vi "Controller Configuration Loop.vi"(7 "Sync Objects":T1, 8 "error in (no error)":errorcluster, 11 "FOFB Configuration":T4={"FOFB Parameters"={"Network"={"FOFB Controller IP"="", "LNLS Control Network IP"="", "LNLS Control Network Power Supplies TCP Port"=0, "LNLS Control Network FOFB Configuration TCP Port"=0, "LNLS Control Network BPMs TCP Port"=0, "Data Server TCP Port"=0, "Monitoring Data TCP Port"=0, "Configuration GUI TCP Port"=0, "Storage Data TCP Port"=0, "Fast Command TCP Port"=0, "TCP Listening Timeout"=0, "Request Setpoints Rate"=0}, "Fast Acquisition"={"Acquisition Period"=0, "Data Buffer Size"=0, "Monitoring Period"=0}, "Response Matrix Measurement"={"Step Amplitude"=0.0, "Time Between Steps"=0, "Step Duration"=0, "Number of Averages"=0}, "Correction Algorithm"={"Correction Period"=0, "Reference Orbit Path"=path "", "Response Matrix Path"=path "", "Correction Matrix Path"=path "", "PID Horizontal Gain"=0.0, "PID Vertical Gain"=0.0, "PID Horizontal Integral Time"=0.0, "PID Vertical Integral Time"=0.0, "PID Horizontal Derivative Time"=0.0, "PID Vertical Derivative Time"=0.0, "Beam Current FOFB Threshold"=0.0, "Decouple H-V"=FALSE, "Use Additional BPM LPF"=FALSE, "BPM LPF Cutoff"=0.0}, "Acquisition Network"=[], "Actuation Network"=[]}, "Number of Acquisition Chassis"=0, "Number of Actuation Chassis"=0, "Number of BPM Readings"=0, "BPM Reading Names"=[], "Selected BPM Readings"=[0, 1, 2, 3, 4, 5, 6, 7, 8, 9, 10, 11, 12, 13, 14, 15, 16, 17, 18, 19, 20, 21, 22, 23, 24, 25, 26, 27, 28, 29, 30, 31, 32, 33, 34, 35, 36, 37, 38, 39, 40, 41, 42, 43, 44, 45, 46, 47, 48, 49], "Number of Correctors"=0, "Corrector Names"=[], "Selected Correctors"=[0, 1, 2, 3, 4, 5, 6, 7, 8, 9, 10, 11, 12, 13, 14, 15, 16, 17, 18, 19, 20, 21, 22, 23, 24, 25, 26, 27, 28, 29, 30, 31, 32, 33, 34, 35, 36, 37, 38, 39, 40, 41, 42, 43, 44, 45, 46, 47, 48, 49], "Reference Orbit"=[], "Response Matrix"=[], "Correction Matrix"=[], "Acquisition Chassis Names"=[], "Actuation Chassis Names"=[], "Acquisition Variables"=[], "Actuation Variables"=[], "PS Matrix Mapping"=[], "Inverse PS Matrix Mapping"=[], "BPM Matrix Mapping"=[], "Inverse BPM Matrix Mapping"=[], "Response Matrix Beam Energy (MeV)"=0.0, "PID Parameters"=[], "BPM Planes"=[], "Corrector Planes"=[], "RMM Step Factor"=[]}) -> (0 "error out":errorcluster)   [LabVIEW 2011, in "Controller VIs.lvlib"]
uses:
  Controller VIs.lvlib
  Types Definitions/Type FOFB Configuration.ctl
  Types Definitions/Type FOFB Parameters.ctl
  Types Definitions/Type Network Configuration.ctl
  Types Definitions/Type FA Configuration.ctl
  Types Definitions/Type Response Matrix Measurement Configuration.ctl
  Types Definitions/Type Correction Algorithm Configuration.ctl
  Types Definitions/Type Acquisition Network Configuration.ctl
  Types Definitions/Type Actuation Network Configuration.ctl
  Types Definitions/Type PID Parameters.ctl
  Types Definitions/Type Synchronization Objects.ctl
  Types Definitions/Type Blocking Synchronization Objects.ctl
  Types Definitions/Type Monitoring Data.ctl
  Types Definitions/Type Operation Mode State.ctl
  Types Definitions/Type Diagnostics Data.ctl
  Types Definitions/Type CPU Loads Array.ctl
  Types Definitions/Type CPU Loads.ctl
  Types Definitions/Type Non-blocking Synchronization Objects.ctl
  Types Definitions/Type FOFB Variables.ctl
  Types Definitions/Type Actuation State.ctl
  Types Definitions/Type TCP State.ctl
  <vilib>/Platform/TimedLoop/XDataNode/timing_clust.ctl
  <vilib>/Platform/TimedLoop/XDataNode/nitl_modes.ctl
  <vilib>/Platform/TimedLoop/XDataNode/wakeup.ctl
  Types Definitions/Type Configuration Data (GUI to Controller).ctl
  Controller Global Variables/LNLS Control FOFB Configuration In.vi
  <vilib>/Platform/TimedLoop/XDataNode/XDataNode.xnode
  Type Definitions.lvlib
  <vilib>/Platform/TimedLoop/XDataNode/XDNodeRunTimeDep.lvlib
  XML VIs.lvlib
  Controller Global Variables.lvlib
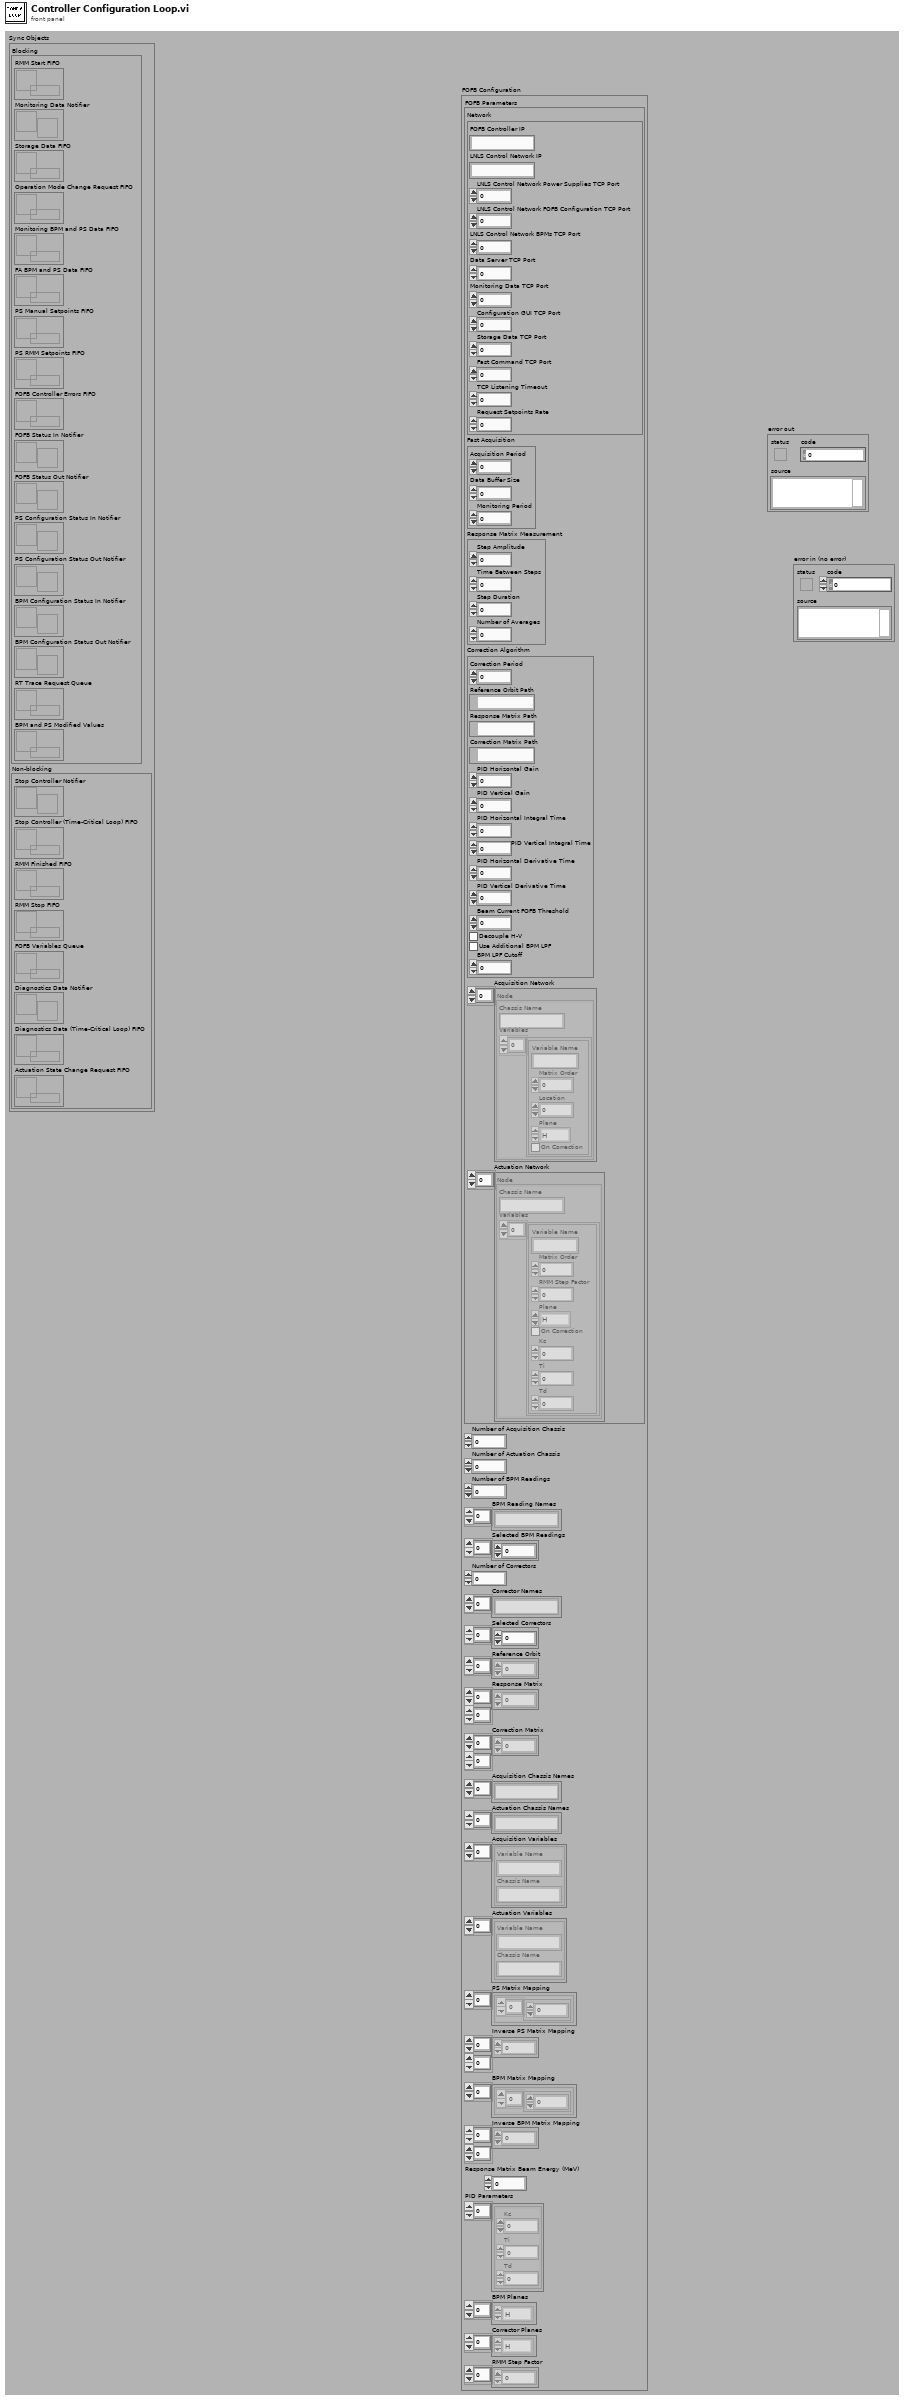
[diagram p1: front panel]
types:
  T1 = typedef "Type Definitions.lvlib/Type Synchronization Objects.ctl" = cluster{"Blocking":T2, "Non-blocking":T3}
  T2 = typedef "Type Definitions.lvlib/Type Blocking Synchronization Objects.ctl" = cluster{"RMM Start FIFO":refnum<k33>, "Monitoring Data Notifier":refnum<notifier>, "Storage Data FIFO":refnum<queue>, "Operation Mode Change Request FIFO":refnum<k33>, "Monitoring BPM and PS Data FIFO":refnum<k33>, "FA BPM and PS Data FIFO":refnum<k33>, "PS Manual Setpoints FIFO":refnum<k33>, "PS RMM Setpoints FIFO":refnum<k33>, "FOFB Controller Errors FIFO ":refnum<k33>, "FOFB Status In Notifier":refnum<notifier>, "FOFB Status Out Notifier":refnum<notifier>, "PS Configuration Status In Notifier":refnum<notifier>, "PS Configuration Status Out Notifier":refnum<notifier>, "BPM Configuration Status In Notifier":refnum<notifier>, "BPM Configuration Status Out Notifier":refnum<notifier>, "RT Trace Request Queue":refnum<queue>, "BPM and PS Modified Values":refnum<k33>}
  T3 = typedef "Type Definitions.lvlib/Type Non-blocking Synchronization Objects.ctl" = cluster{"Stop Controller Notifier":refnum<notifier>, "Stop Controller (Time-Critical Loop) FIFO":refnum<k33>, "RMM Finished FIFO":refnum<k33>, "RMM Stop FIFO":refnum<k33>, "FOFB Variables Queue":refnum<queue>, "Diagnostics Data Notifier":refnum<notifier>, "Diagnostics Data (Time-Critical Loop) FIFO":refnum<k33>, "Actuation State Change Request FIFO":refnum<k33>}
  T4 = typedef "Type Definitions.lvlib/Type FOFB Configuration.ctl" = cluster{"FOFB Parameters":T5, "Number of Acquisition Chassis":i32, "Number of Actuation Chassis":i32, "Number of BPM Readings":i32, "BPM Reading Names":string[], "Selected BPM Readings":u32[], "Number of Correctors":i32, "Corrector Names":string[], "Selected Correctors":u32[], "Reference Orbit":dbl[], "Response Matrix":dbl[][], "Correction Matrix":dbl[][], "Acquisition Chassis Names":string[], "Actuation Chassis Names":string[], "Acquisition Variables":cluster{"Variable Name":string, "Chassis Name":string}[], "Actuation Variables":cluster{"Variable Name":string, "Chassis Name":string}[], "PS Matrix Mapping":cluster{u32[]}[], "Inverse PS Matrix Mapping":u32[][], "BPM Matrix Mapping":cluster{u32[]}[], "Inverse BPM Matrix Mapping":u32[][], "Response Matrix Beam Energy (MeV)":dbl, "PID Parameters":T12[], "BPM Planes":enum8{"H", "V"}[], "Corrector Planes":enum8{"H", "V"}[], "RMM Step Factor":dbl[]}
  T5 = typedef "Type Definitions.lvlib/Type FOFB Parameters.ctl" = cluster{"Network":T6, "Fast Acquisition":T7, "Response Matrix Measurement":T8, "Correction Algorithm":T9, "Acquisition Network":T10, "Actuation Network":T11}
  T6 = typedef "Type Definitions.lvlib/Type Network Configuration.ctl" = cluster{"FOFB Controller IP":string, "LNLS Control Network IP":string, "LNLS Control Network Power Supplies TCP Port":u16, "LNLS Control Network FOFB Configuration TCP Port":u16, "LNLS Control Network BPMs TCP Port":u16, "Data Server TCP Port":u16, "Monitoring Data TCP Port":u16, "Configuration GUI TCP Port":u16, "Storage Data TCP Port":u16, "Fast Command TCP Port":u16, "TCP Listening Timeout":i32, "Request Setpoints Rate":u16}
  T7 = typedef "Type Definitions.lvlib/Type FA Configuration.ctl" = cluster{"Acquisition Period":u32, "Data Buffer Size":u32, "Monitoring Period":u32}
  T8 = typedef "Type Definitions.lvlib/Type Response Matrix Measurement Configuration.ctl" = cluster{"Step Amplitude":dbl, "Time Between Steps":u32, "Step Duration":u32, "Number of Averages":u32}
  T9 = typedef "Type Definitions.lvlib/Type Correction Algorithm Configuration.ctl" = cluster{"Correction Period":u32, "Reference Orbit Path":path, "Response Matrix Path":path, "Correction Matrix Path":path, "PID Horizontal Gain":dbl, "PID Vertical Gain":dbl, "PID Horizontal Integral Time":dbl, "PID Vertical Integral Time":dbl, "PID Horizontal Derivative Time":dbl, "PID Vertical Derivative Time":dbl, "Beam Current FOFB Threshold":dbl, "Decouple H-V":bool, "Use Additional BPM LPF":bool, "BPM LPF Cutoff":dbl}
  T10 = typedef "Type Definitions.lvlib/Type Acquisition Network Configuration.ctl" = cluster{"Chassis Name":string, "Variables":cluster{"Variable Name":string, "Matrix Order":u32, "Location":dbl, "Plane":enum8{"H", "V"}, "On Correction":bool}[]}[]
  T11 = typedef "Type Definitions.lvlib/Type Actuation Network Configuration.ctl" = cluster{"Chassis Name":string, "Variables":cluster{"Variable Name":string, "Matrix Order":u32, "RMM Step Factor":dbl, "Plane":enum8{"H", "V"}, "On Correction":bool, "Kc":dbl, "Ti":dbl, "Td":dbl}[]}[]
  T12 = typedef "Type Definitions.lvlib/Type PID Parameters.ctl" = cluster{"Kc":fxp<+/-,16,8>, "Ti":fxp<+/-,16,8>, "Td":fxp<+/-,16,8>}
  T13 = typedef "Type Definitions.lvlib/Type TCP State.ctl" = enum16{"Idle", "Wait Connection", "Read Data", "Process Data", "Write Data", "Close Connection"}
  T14 = typedef "XDNodeRunTimeDep.lvlib/timing_clust.ctl" = cluster{"Expected End [f-1]":u64, "Actual End [f-1]":u64, "Finished Late? [f-1]":bool, "Expected End [i-1]":u64, "Actual End [i-1]":u64, "Finished Late? [i-1]":bool, "Expected Start [i]":u64, "Actual Start [i]":u64, "Expected Start [f]":u64, "Actual Start [f]":u64, "Source Name":string, "Structure Name":string, "Period":i64, "Deadline":i64, "Offset":i64, "Start":i64, "Priority":i32, "Timeout":i32, "Mode":T15, "Wakeup Reason":T16, "Error":errorcluster, "Source Type":string, "Secondary Source Type":string, "Global End Time":u64, "Global Start Time":u64, "Frame Duration":u64, "Iteration Duration":u64, "Assigned CPU":i32, "I/O Scan Engine Mode":u32}
  T15 = typedef "XDNodeRunTimeDep.lvlib/nitl_modes.ctl" = enum32{"No Change", "Process missed periods, maintain original phase", "Discard missed periods, maintain original phase", "Process missed periods, ignore original phase", "Discard missed periods, ignore original phase"}
  T16 = typedef "XDNodeRunTimeDep.lvlib/wakeup.ctl" = enum32{"Normal", "Aborted", "Asynchronous wakeup", "Timing source error", "Timed loop error", "Timeout"}
  T17 = typedef "Type Definitions.lvlib/Type Configuration Data (GUI to Controller).ctl" = cluster{"Update Controller Soft Configuration":bool[], "Request RT Execution Trace":string[], "Reference Orbit":dbl[], "Request Response Matrix Folder List":bool[], "Request FOFB Parameters":bool[], "FOFB Parameters":T5[]}
  T18 = typedef "Type Definitions.lvlib/Type Configuration Change Acknowledge (Controller to GUI).ctl" = cluster{"Request Response Matrix List Folder":string[], "FOFB Parameters":T5[]}
  T19 = typedef "Type Definitions.lvlib/Type Control FOFB Configuration In.ctl" = cluster{"Status":u16, "Operation Mode":T20, "PID Horizontal Gain":sgl, "PID Vertical Gain":sgl, "PID Horizontal Integral Time":sgl, "PID Vertical Integral Time":sgl, "PID Horizontal Derivative Time":sgl, "PID Vertical Derivative Time":sgl, "Fast Command Enabled":bool}
  T20 = typedef "Type Definitions.lvlib/Type Operation Mode State.ctl" = enum8{"Idle Mode", "Manual Mode", "FOFB Mode", "RMM Mode"}
  T21 = cluster{"PID Horizontal Gain":sgl, "PID Vertical Gain":sgl, "PID Horizontal Integral Time":sgl, "PID Vertical Integral Time":sgl, "PID Horizontal Derivative Time":sgl, "PID Vertical Derivative Time":sgl, "Fast Command Enabled":bool}
  T22 = typedef "Type Definitions.lvlib/Type FOFB Variables.ctl" = cluster{"Correction Period":u32, "Reference Orbit":dbl[], "Response Matrix":dbl[][], "Correction Matrix":dbl[][], "Decouple H-V":bool, "PID Horizontal Gain":dbl, "PID Vertical Gain":dbl, "PID Horizontal Integral Time":dbl, "PID Vertical Integral Time":dbl, "PID Horizontal Derivative Time":dbl, "PID Vertical Derivative Time":dbl, "Selected BPM Readings":u32[], "Selected Correctors":u32[], "BPM Planes":enum8{"H", "V"}[], "Corrector Planes":enum8{"H", "V"}[], "Beam Current FOFB Threshold":dbl, "Response Matrix Beam Energy (MeV)":dbl, "Fast Command Enabled":bool}
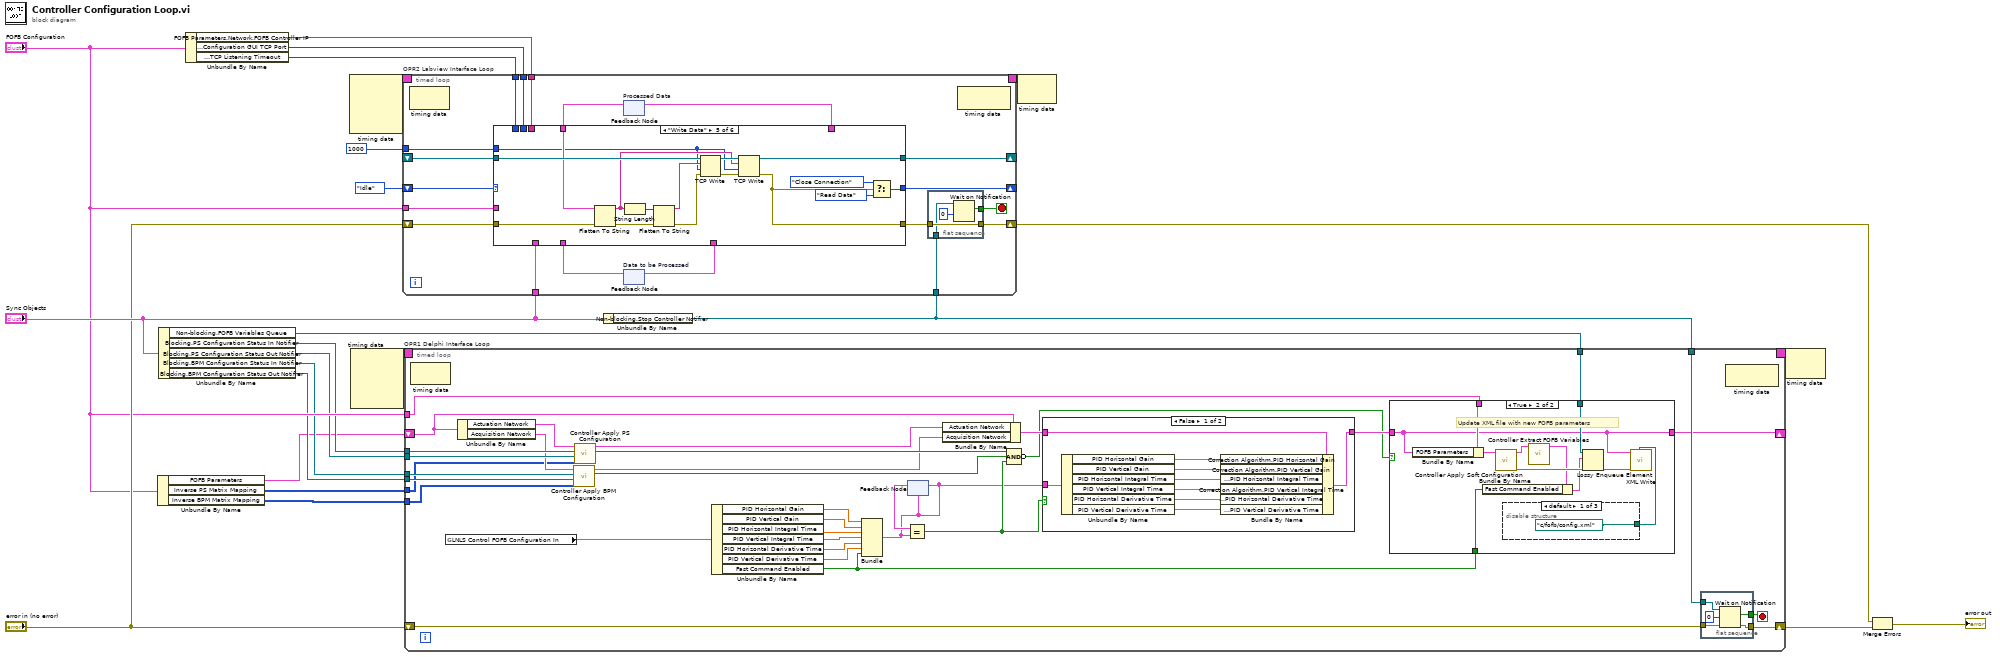
[diagram p0: block diagram]
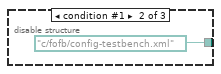
[diagram p4: hidden frame]
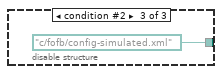
[diagram p5: hidden frame]
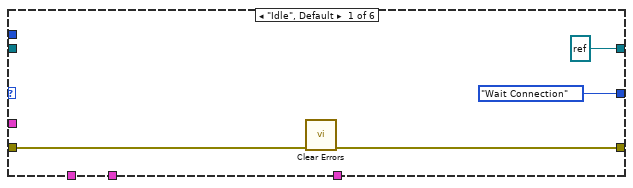
[diagram p6: hidden frame]
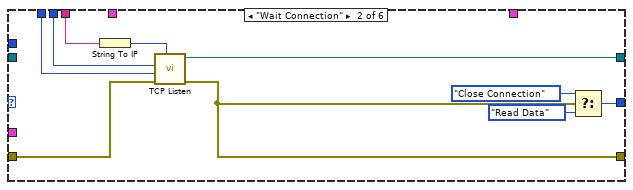
[diagram p7: hidden frame]
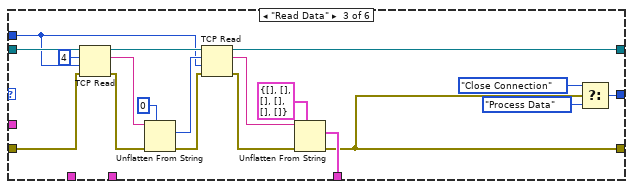
[diagram p8: hidden frame]
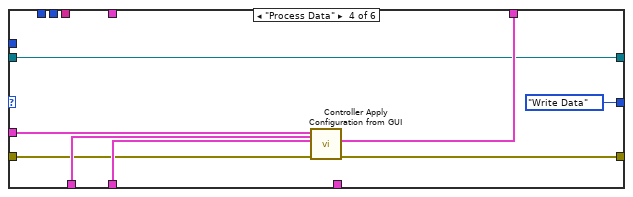
[diagram p9: hidden frame]
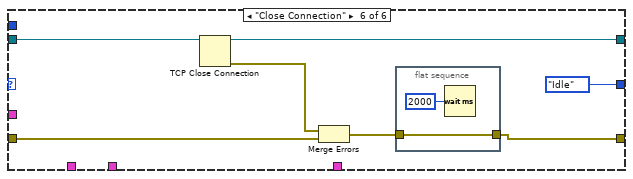
[diagram p10: hidden frame]
diagram:
  n1 = Unbundle By Name("FOFB Configuration") -> ("FOFB Parameters"=w4:T5, "Inverse PS Matrix Mapping"=w3:u32[][], "Inverse BPM Matrix Mapping"=w2:u32[][])
  n2 = Unbundle By Name("Sync Objects") -> ("Non-blocking.FOFB Variables Queue"=w9:refnum<queue>, "Blocking.PS Configuration Status In Notifier"=w7:refnum<notifier>, "Blocking.PS Configuration Status Out Notifier"=w6:refnum<notifier>, "Blocking.BPM Configuration Status In Notifier"=w8:refnum<notifier>, "Blocking.BPM Configuration Status Out Notifier"=w5:refnum<notifier>)
  n3 = Unbundle By Name("FOFB Configuration") -> ("FOFB Parameters.Network.FOFB Controller IP"=w24:string, "FOFB Parameters.Network.Configuration GUI TCP Port"=w22:u16, "FOFB Parameters.Network.TCP Listening Timeout"=w23:i32)
  n4 = node-c288() -> (w21:T14)  [unwired: 4 in]
  n5 = node-c288() -> (w11:T14)  [unwired: 4 in]
  n6 = Unbundle By Name("Sync Objects") -> ("Non-blocking.Stop Controller Notifier"=w17:refnum<notifier>)
  n7 = timed-loop "OPR2 Labview Interface Loop" {
    tunnel: w24 -> [w43]
    tunnel: w22 -> [w42]
    tunnel: w23 -> [w41]
    shift-right: [w29] -> w15
    shift-left: "error in (no error)" -> [w38]
    shift-right: [w36] -> _
    shift-left: Type_TCP_State."Idle" ("f") -> [w37]
    shift-right: [w39] -> _
    shift-left: _ -> [w40]
    tunnel: w17 -> [w28]
    tunnel: "Sync Objects" -> [w33]
    timing: w21 -> [_]
    timing-out: [_] -> w20
    tunnel: "FOFB Configuration" -> [w26]
    tunnel: 1000 ("TCP Listening Timeout") -> [w25]
    stop <- w27 stop-if-true
    n8 = node-c288() -> ()  [unwired: 1 in, 1 out]
    n9 = feedback #1 "Processed Data"() -> (w32:T18)  [unwired: 1 in]
    n10 = feedback #2 "Data to be Processed"() -> (w34:T17)  [unwired: 1 in]
    n11 = case shown="\"Write Data\"" w37 {
      tunnel: [refnum<k5> refnum ("connection ID") w63 w75 w89 w106 w113] -> w39
      tunnel: [Type_TCP_State."Wait Connection" ("f") w62 w71 Type_TCP_State."Write Data" ("f") w105 Type_TCP_State."Idle" ("f")] -> w36
      tunnel: [w50 w57 w67 w83 w104 w107] -> w30
      tunnel: w38 -> [w51 w56 w74 w84 w94 w109]
      tunnel: w40 -> [_ _ w76 w89 w102 w111]
      tunnel: w43 -> [_ w61 _ _ _ _]
      tunnel: w42 -> [_ w59 _ _ _ _]
      tunnel: w41 -> [_ w54 _ _ _ _]
      tunnel: [_ _ w69 _ _ _] -> w35
      tunnel: w34 -> [_ _ _ w86 _ _]
      tunnel: w33 -> [_ _ _ w87 _ _]
      tunnel: w32 -> [_ _ _ _ w95 _]
      tunnel: [_ _ _ w90 _ _] -> w31
      tunnel: w26 -> [_ _ _ w85 _ _]
      tunnel: w25 -> [_ _ w64 _ w91 _]
      frame "Idle", Default {
        n12 = call <vilib>:"Clear Errors.vi"("error in (no error)"=w51) -> ("error out"=w50:errorcluster)  [unwired: 6 in]
      }
      frame "Wait Connection" {
        n13 = String To IP(1:w61) -> (0:w60:u32)
        n14 = call <vilib>:"TCP Listen.vi"("net address"=w60, "error in (no error)"=w56, "timeout ms (wait forever: -1)"=w54, "port"=w59) -> ("error out"=w57:errorcluster, "connection ID"=w63:refnum<k5>)  [unwired: 3 in, 3 out]
        n15 = Select(t=Type_TCP_State."Close Connection" ("f"), s=w57, f=Type_TCP_State."Read Data") -> (s? t:f=w62:T13)
      }
      frame "Read Data" {
        n16 = TCP Read(connection ID=w76, bytes to read=4, error in (no error)=w74, 9:w64) -> (connection ID out=w82:refnum<k5>, data out=w80:string, error out=w66:errorcluster)  [unwired: 1 in]
        n17 = Unflatten From String(type=0 ("bytes to read"), binary string=w80, error in (no error)=w66) -> (value=w78:i32, error out=w68:errorcluster)  [unwired: 2 in, 1 out]
        n18 = TCP Read(connection ID=w82, bytes to read=w78, error in (no error)=w68, 9:w64) -> (connection ID out=w75:refnum<k5>, data out=w77:string, error out=w65:errorcluster)  [unwired: 1 in]
        n19 = Unflatten From String(type=T17 {"Update Controller Soft Configuration"=[], "Request RT Execution Trace"=[], "Reference Orbit"=[], "Request Response Matrix Folder List"=[], "Request FOFB Parameters"=[], "FOFB Parameters"=[]} ("Configuration Data (GUI to Controller)"), binary string=w77, error in (no error)=w65) -> (value=w69:T17, error out=w67:errorcluster)  [unwired: 2 in, 1 out]
        n20 = Select(t=Type_TCP_State."Close Connection" ("f"), s=w67, f=Type_TCP_State."Process Data") -> (s? t:f=w71:T13)
      }
      frame "Process Data" {
        n21 = call "Controller Apply Configuration from GUI.vi"("Sync Objects"=w87, "error in (no error)"=w84, "Configuration Data (GUI to Controller)"=w86, "FOFB Configuration"=w85) -> ("error out"=w83:errorcluster, "Configuration Change Acknowledge (Controller to GUI)"=w90:T18)  [unwired: 6 in]
      }
      frame "Write Data" {
        n22 = Flatten To String(anything=w95, error in (no error)=w94) -> (data string=w98:string, error out=w93:errorcluster)  [unwired: 2 in, 1 out]
        n23 = String Length(string=w98) -> (length=w100:i32)
        n24 = Flatten To String(anything=w100, error in (no error)=w93) -> (data string=w99:string, error out=w92:errorcluster)  [unwired: 2 in, 1 out]
        n25 = TCP Write(connection ID=w102, data in=w99, error in (no error)=w92, 9:w91) -> (connection ID out=w103:refnum<k5>, error out=w101:errorcluster)  [unwired: 1 out]
        n26 = TCP Write(connection ID=w103, data in=w98, error in (no error)=w101, 9:w91) -> (connection ID out=w106:refnum<k5>, error out=w104:errorcluster)  [unwired: 1 out]
        n27 = Select(t=Type_TCP_State."Close Connection" ("f"), s=w104, f=Type_TCP_State."Read Data") -> (s? t:f=w105:T13)
      }
      frame "Close Connection" {
        n28 = TCP Close Connection(connection ID=w111) -> (connection ID out=w113:refnum<k5>, error out=w110:errorcluster)  [unwired: 2 in]
        n29 = Merge Errors(w110, w109) -> (w108:errorcluster)
        n30 = flat-sequence {
          tunnel: w108 -> [w114]
          tunnel: [w114] -> w107
          frame #0 {
            n31 = Wait (ms)(milliseconds to wait=u32 2000) -> ()  [unwired: 1 out]
          }
        }
      }
    }
    n32 = feedback-in #1(w31) -> ()
    n33 = feedback-in #2(w35) -> ()
    n34 = flat-sequence {
      tunnel: [w48] -> w27
      tunnel: w30 -> [w47]
      tunnel: [w47] -> w29
      tunnel: w28 -> [w46]
      frame #0 {
        n35 = Wait on Notification(notifier=w46, timeout in ms (-1)=0) -> (notification=w48:bool)  [unwired: 2 in, 3 out]
      }
    }
    n36 = node-c288() -> ()  [unwired: 1 in, 1 out]
  }
  n37 = timed-loop "OPR1 Delphi Interface Loop" {
    timing: w11 -> [_]
    timing-out: [_] -> w10
    tunnel: w7 -> [w142]
    shift-right: [w141] -> _
    shift-left: w4 -> [w149]
    tunnel: w9 -> [w148]
    tunnel: "FOFB Configuration" -> [w147]
    tunnel: w17 -> [w143]
    shift-right: [w144] -> w13
    shift-left: "error in (no error)" -> [w145]
    tunnel: w8 -> [w136]
    tunnel: w6 -> [w137]
    tunnel: w5 -> [w134]
    tunnel: w3 -> [w131]
    tunnel: w2 -> [w130]
    stop <- w146 stop-if-true
    n38 = node-c288() -> ()  [unwired: 1 in, 1 out]
    n39 = global read "LNLS Control FOFB Configuration In.vi" "LNLS Control FOFB Configuration In"() -> (w117:T19)
    n40 = Unbundle By Name(w149) -> ("Actuation Network"=w133:T11, "Acquisition Network"=w135:T10)
    n41 = call "Controller Apply BPM Configuration.vi"("Inverse BPM Matrix Mapping"=w130, "BPM Configuration Status Out"=w134, "BPM Configuration Status In"=w136, "Acquisition Network In"=w135) -> ("Maintain Config?"=w138:bool, "Acquisition Network Out"=w139:T10)  [unwired: 6 in]
    n42 = call "Controller Apply PS Configuration.vi"("Inverse PS Matrix Mapping"=w131, "PS Configuration Status Out"=w137, "PS Configuration Status In"=w142, "Actuation Network In"=w133) -> ("Maintain Config?"=w140:bool, "Actuation Network Out"=w132:T11)  [unwired: 6 in]
    n43 = Unbundle By Name(w117) -> ("PID Horizontal Gain"=w120:sgl, "PID Vertical Gain"=w121:sgl, "PID Horizontal Integral Time"=w122:sgl, "PID Vertical Integral Time"=w123:sgl, "PID Horizontal Derivative Time"=w118:sgl, "PID Vertical Derivative Time"=w124:sgl, "Fast Command Enabled"=w116:bool)
    n44 = Bundle("PID Horizontal Gain"=w120, "PID Vertical Gain"=w121, "PID Horizontal Integral Time"=w122, "PID Vertical Integral Time"=w123, "PID Horizontal Derivative Time"=w118, "PID Vertical Derivative Time"=w124, "Fast Command Enabled"=w116) -> (w119:T21)  [unwired: 1 in]
    n45 = feedback-in #3(w119) -> ()
    n46 = feedback #3(w119) -> (w129:T21)
    n47 = Equal?(x=w129, y=w119) -> (x = y?=w125:bool)
    n48 = Bundle By Name(cluster=w149, "Actuation Network"=w132, "Acquisition Network"=w139) -> (w127:T5)
    n49 = Compound Arithmetic op=AND(w140, w138, w125) -> (invert w126:bool)
    n50 = case shown="False" w125 {
      tunnel: w127 -> [w158 w159]
      tunnel: [w157 w159] -> w128
      tunnel: w119 -> [w156 _]
      frame False {
        n51 = Unbundle By Name(w156) -> ("PID Horizontal Gain"=w155:sgl, "PID Vertical Gain"=w154:sgl, "PID Horizontal Integral Time"=w153:sgl, "PID Vertical Integral Time"=w152:sgl, "PID Horizontal Derivative Time"=w151:sgl, "PID Vertical Derivative Time"=w150:sgl)
        n52 = Bundle By Name(cluster=w158, "Correction Algorithm.PID Horizontal Gain"=w155, "Correction Algorithm.PID Vertical Gain"=w154, "Correction Algorithm.PID Horizontal Integral Time"=w153, "Correction Algorithm.PID Vertical Integral Time"=w152, "Correction Algorithm.PID Horizontal Derivative Time"=w151, "Correction Algorithm.PID Vertical Derivative Time"=w150) -> (w157:T5)
      }
      frame True {
      }
    }
    n53 = case shown="True" w126 {
      tunnel: w148 -> [_ w171]
      tunnel: w147 -> [_ w170]
      tunnel: w128 -> [w160 w165]
      tunnel: [w160 w165] -> w141
      tunnel: w116 -> [_ w163]
      frame False {
      }
      frame True {
        # "Update XML file with new FOFB parameters"
        n54 = Bundle By Name(cluster=w170, "FOFB Parameters"=w165) -> (w164:T4)
        n55 = call "Controller Apply Soft Configuration.vi"("FOFB Configuration"=w164) -> ("error out"=w168:errorcluster, "FOFB Configuration"=w169:T4)  [unwired: 9 in]
        n56 = disable-structure shown="default" {
          disable-tunnel: [path "c:/fofb/config.xml" ("Configuration File Path") path "c:/fofb/config-testbench.xml" ("Configuration File Path") path "c:/fofb/config-simulated.xml" ("Configuration File Path")] -> w166
          frame condition #0 (active) {
          }
          frame condition #1 {
          }
          frame condition #2 {
          }
        }
        n57 = call "Controller Extract FOFB Variables.vi"("FOFB Configuration"=w169) -> ("FOFB Variables"=w162:T22)  [unwired: 9 in, 1 out]
        n58 = Bundle By Name(cluster=w162, "Fast Command Enabled"=w163) -> (w161:T22)
        n59 = Lossy Enqueue Element(queue=w171, element=w161, error in (no error)=w168) -> (error out=w167:errorcluster)  [unwired: 3 out]
        n60 = call "XML Write.vi"("XML File Path Write"=w166, "Error In"=w167, "FOFB Parameters"=w165) -> ()  [unwired: 7 in, 2 out]
      }
    }
    n61 = flat-sequence {
      tunnel: [w178] -> w146
      tunnel: w143 -> [w177]
      tunnel: w145 -> [w176]
      tunnel: [w175] -> w144
      frame #0 {
        n62 = Wait on Notification(notifier=w177, timeout in ms (-1)=0, error in (no error)=w176) -> (notification=w178:bool, error out=w175:errorcluster)  [unwired: 1 in, 2 out]
      }
    }
    n63 = node-c288() -> ()  [unwired: 1 in, 1 out]
  }
  n64 = node-c288(w20) -> ()  [unwired: 1 out]
  n65 = node-c288(w10) -> ()  [unwired: 1 out]
  n66 = Merge Errors(w15, w13) -> (→"error out":errorcluster)
